vi "AIT 1553 - Parse BM Channels.vi"(6 "Bus Config Info":T12, 7 "FIFO Idx Qs":T14, 8 "error in (no error)":errorcluster, 10 "Section GUID":string, 11 "Device Reference in":T15 format="%.0x") -> (0 "error out":errorcluster, 1 "Section BaseRate":u32, 2 "HW Channel - BM Section":T1 {"Message Settings"."Driver Data"."First Word" min=8 max=31; "Message Settings"."Driver Data"."Num Bits" min=1 max=32; "Message Settings"."Driver Data"."Start Bit" min=8 max=31; "Message Settings"."Block Data Refs"."Data Reference" format="%.0x"; "Rx Com Udp Port"."Handle" format="%08x"; "Tx Com Udp Port"."Handle" format="%08x"}, 3 "Device Reference out":T15 format="%.0x")   [LabVIEW 2013]
uses:
  <vilib>/NI Veristand/Custom Device Tools/Custom Device Utility Library/Custom Device Utility Library.lvlib
  <vilib>/NI Veristand/Custom Device API/Custom Device API.lvlib
  Controls and Global/Number of Bits.ctl
  AIT 664 Custom Device.lvlib
  Controls and Global/Start Bit.ctl
  <vilib>/NI Veristand/Custom Device API/Data Reference.ctl
  <vilib>/NI Veristand/Custom Device API/Block Data Reference.ctl
  Controls and Global/Global.vi
  <vilib>/NI Veristand/Custom Device Tools/Custom Device Utility Library/NI VeriStand - Search for Item by GUID.vi
  RT Controls/AIT 664 - RT Message Settings.ctl
  RT Controls/AIT 664 - RT Hardware Channel.ctl
  RT Controls/AIT 664 - Driver Data.ctl
  RT Controls/AIT 1553 - Bus Section.ctl
  System Explorer/Controls/664 - Sampling Type.ctl
  <userlib>/ARINC 664/AIT 664 Controls/General/Message Port Type.ctl
  <userlib>/ARINC 664/AIT 664 API.lvlib
  <userlib>/ARINC 664/AIT 664 Controls/General/Direction.ctl
  <userlib>/ARINC 664/AIT 664 Controls/General/Message Port.ctl
  <vilib>/NI Veristand/Custom Device API/Custom Device Item Ref.ctl
  RT Controls/FIFO Index Queues.ctl
  RT Controls/AIT 1553 - Hardware Type.ctl
  RT Controls/AIT 1553 - Board Config Info.ctl
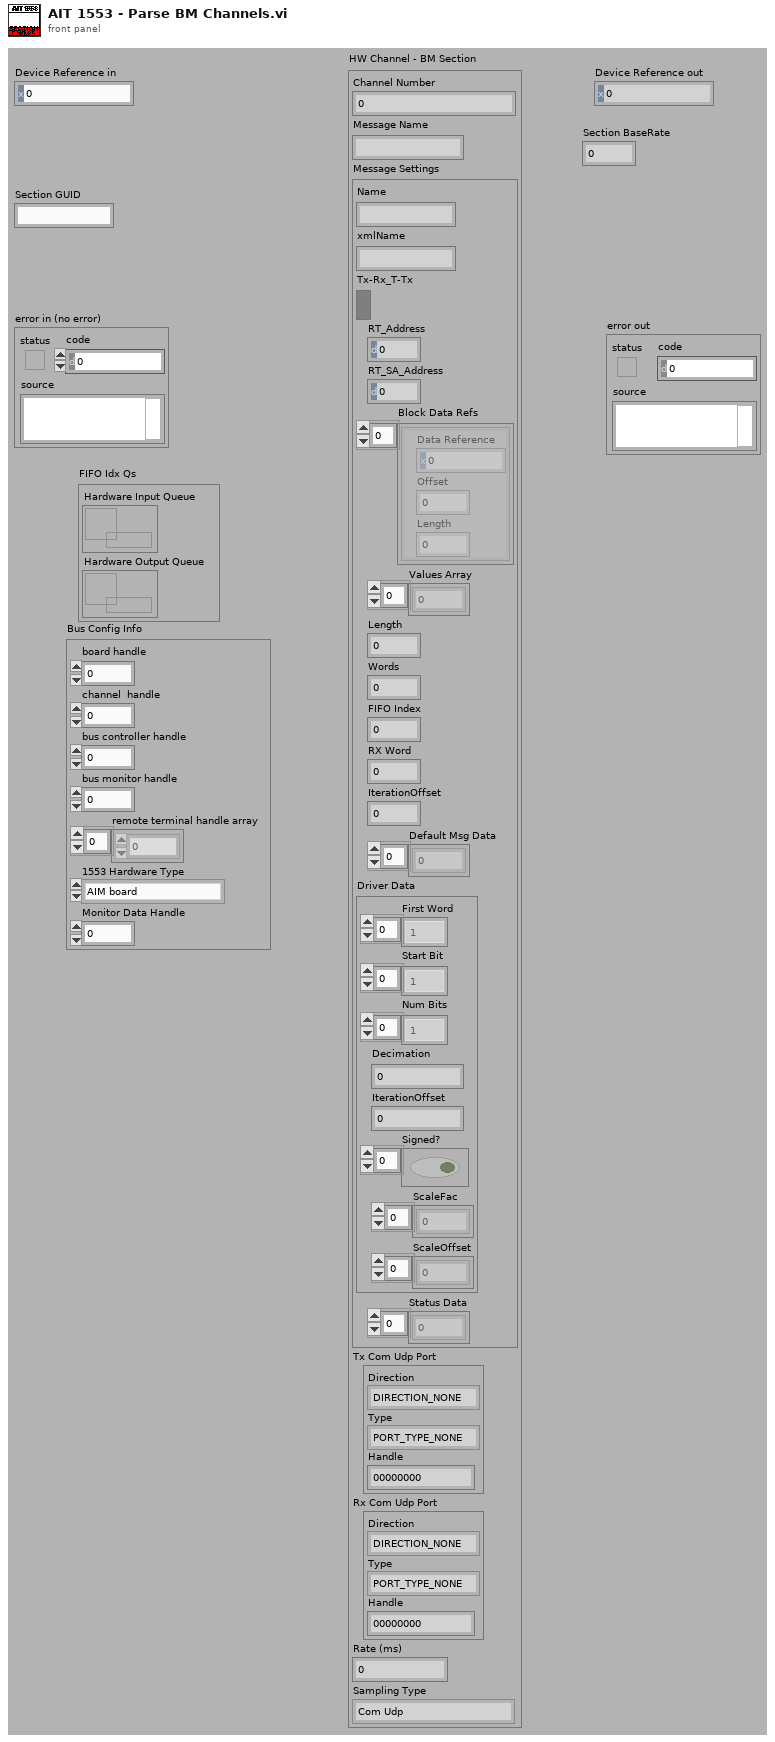
[diagram p1: front panel]
types:
  T1 = typedef "AIT 664 Custom Device.lvlib/AIT 664 - RT Hardware Channel.ctl" = cluster{"Channel Number":u16, "Message Name":string, "Message Settings":T2, "Tx Com Udp Port":T8, "Rx Com Udp Port":T8, "Rate (ms)":u32, "Sampling Type":T11}
  T2 = typedef "AIT 664 Custom Device.lvlib/AIT 664 - RT Message Settings.ctl" = cluster{"Name":string, "xmlName":string, "Tx-Rx_T-Tx":bool, "RT_Address":u8, "RT_SA_Address":u8, "Block Data Refs":T3[], "Values Array":dbl[], "Length":i32, "Words":i32, "FIFO Index":i32, "RX Word":u32, "IterationOffset":i32, "Default Msg Data":u8[], "Driver Data":T5, "Status Data":u32[]}
  T3 = typedef "Custom Device API.lvlib/Block Data Reference.ctl" = cluster{"Data Reference":T4, "Offset":i32, "Length":i32}
  T4 = typedef "Custom Device API.lvlib/Data Reference.ctl" = i32
  T5 = typedef "AIT 664 Custom Device.lvlib/AIT 664 - Driver Data.ctl" = cluster{"First Word":T6[], "Start Bit":T6[], "Num Bits":T7[], "Decimation":i32, "IterationOffset":i32, "Signed?":bool[], "ScaleFac":dbl[], "ScaleOffset":dbl[]}
  T6 = typedef "AIT 664 Custom Device.lvlib/Start Bit.ctl" = i32
  T7 = typedef "AIT 664 Custom Device.lvlib/Number of Bits.ctl" = i32
  T8 = typedef "AIT 664 API.lvlib/Message Port.ctl" = cluster{"Direction":T9, "Type":T10, "Handle":u64}
  T9 = typedef "AIT 664 API.lvlib/Direction.ctl" = enum16{"DIRECTION_NONE", "DIRECTION_TX", "DIRECTION_RX"}
  T10 = typedef "AIT 664 API.lvlib/Message Port Type.ctl" = enum16{"PORT_TYPE_NONE", "COM_UDP", "SAP_UDP", "SAP_IP", "SAP_MAC", "COTS_MAC", "COTS_MAC_RAW"}
  T11 = typedef "AIT 664 Custom Device.lvlib/664 - Sampling Type.ctl" = enum16{"Com Udp", "Com Udp Queuing", "Sap Udp", "Sap Ip", "Sap Mac", "Unknown"}
  T12 = typedef "AIT 1553 - Board Config Info.ctl" = cluster{"board handle":u32, "channel  handle":u32, "bus controller handle":u32, "bus monitor handle":u32, "remote terminal handle array":u32[], "1553 Hardware Type":T13, "Monitor Data Handle":u32}
  T13 = typedef "AIT 1553 - Hardware Type.ctl" = enum16{"AIM board", "AIT Board"}
  T14 = typedef "AIT 664 Custom Device.lvlib/FIFO Index Queues.ctl" = cluster{"Hardware Input Queue":refnum<queue>, "Hardware Output Queue":refnum<queue>}
  T15 = typedef "Custom Device API.lvlib/Custom Device Item Ref.ctl" = u64
  T16 = typedef "AIT 1553 - Bus Section.ctl" = enum16{"BC", "BM", "RT"}
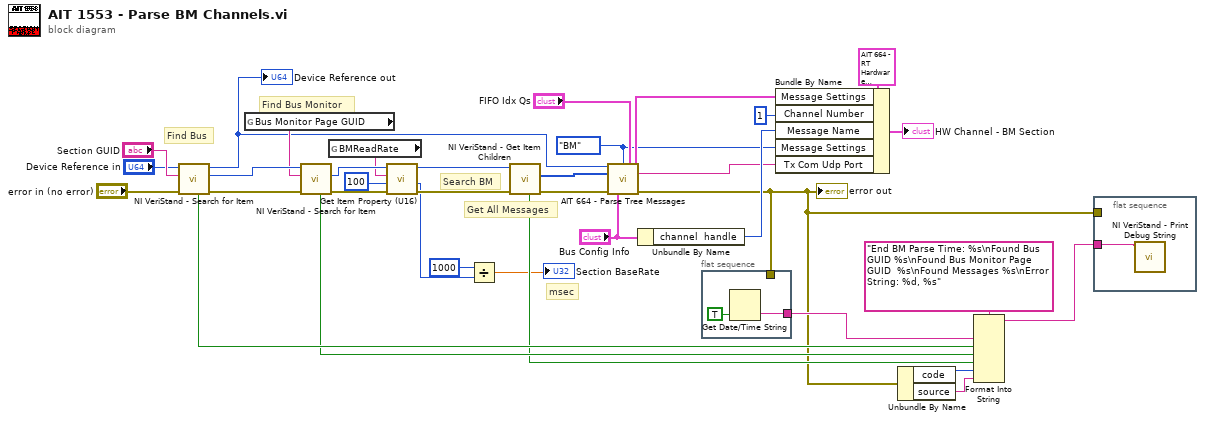
[diagram p0: block diagram]
diagram:
  w15 = AIT_1553_-_Bus_Section."BM" ("Bus Section")
  # "msec"
  # "Find Bus Monitor"
  # "Find Bus"
  # "Get All Messages"
  # "Search BM"
  n1 = call-poly <vilib>:"NI VeriStand - Search for Item.vi"("error in"="error in (no error)", "Item GUID"="Section GUID", "Section Ref in"="Device Reference in") -> ("error out"=w26:errorcluster, "Item Ref"=w27:T15, "Section Ref out"=w16:T15, "Found"=w23:bool)  [unwired: 5 in]
  "Device Reference out" <- w16
  n2 = global read "Global.vi" "Bus Monitor Page GUID"() -> (w25:string)
  n3 = call-poly <vilib>:"NI VeriStand - Search for Item.vi"("error in"=w26, "Item GUID"=w25, "Section Ref in"=w27) -> ("error out"=w9:errorcluster, "Item Ref"=w8:T15, "Found"=w22:bool)  [unwired: 5 in, 1 out]
  n4 = global read "Global.vi" "BMReadRate"() -> (w1:string)
  n5 = call <vilib>:"Get Item Property (U16).vi"("error in (no error)"=w9, "Default Value"=u16 100 ("Section BaseRate"), "Property Name"=w1, "Item Ref in"=w8) -> ("error out"=w6:errorcluster, "Value"=w3:u16, "Item Ref out"=w7:T15)  [unwired: 4 in, 1 out]
  n6 = Divide(x=u16 1000 ("Section BaseRate"), y=w3) -> (x/y=→"Section BaseRate":dbl)
  n7 = call <vilib>:"NI VeriStand - Get Item Children.vi"("error in (no error)"=w6, "Item Ref in"=w7) -> ("error out"=w20:errorcluster, "Child Refs"=w33:T15[], "Found"=w18:bool)  [unwired: 6 in, 1 out]
  n8 = call "AIT 664 - Parse Tree Messages.vi"("Custom Device Ref"=w16, 2:w15, "FIFO Idx Qs"="FIFO Idx Qs", "Message Ref"=w33, "error out"=w20, 12:"Bus Config Info") -> ("Message Settings"=w30:T2, "Message Name"=w14:string, "error out"=w12:errorcluster)  [unwired: 7 in]
  "error out" <- w12
  n9 = Unbundle By Name("Bus Config Info") -> ("channel  handle"=w28:u32)
  n10 = flat-sequence {
    tunnel: [w38] -> w13
    tunnel: w12 -> [_]
    frame #0 {
      n11 = Get Date/Time String(want seconds? (F)=TRUE) -> (time string=w38:string)  [unwired: 2 in, 1 out]
    }
  }
  n12 = Bundle By Name(cluster=T1 {"Channel Number"=0, "Message Name"="", "Message Settings"={"Name"="", "xmlName"="", "Tx-Rx_T-Tx"=FALSE, "RT_Address"=0, "RT_SA_Address"=0, "Block Data Refs"=[], "Values Array"=[], "Length"=0, "Words"=0, "FIFO Index"=0, "RX Word"=0, "IterationOffset"=0, "Default Msg Data"=[], "Driver Data"={"First Word"=[], "Start Bit"=[], "Num Bits"=[], "Decimation"=0, "IterationOffset"=0, "Signed?"=[], "ScaleFac"=[], "ScaleOffset"=[]}, "Status Data"=[]}, "Tx Com Udp Port"={"Direction"=enum."DIRECTION_NONE", "Type"=enum."PORT_TYPE_NONE", "Handle"=0}, "Rx Com Udp Port"={"Direction"=enum."DIRECTION_NONE", "Type"=enum."PORT_TYPE_NONE", "Handle"=0}, "Rate (ms)"=0, "Sampling Type"=enum."Com Udp"} ("HW Channel"), "Message Settings"=w30, "Channel Number"=u16 1 ("channel #"), "Message Name"=w28, "Message Settings"=w15, "Tx Com Udp Port"=w14) -> (→"HW Channel - BM Section":T1)
  n13 = Unbundle By Name(w12) -> ("code"=w19:i32, "source"=w11:string)
  n14 = Format Into String(format string="End BM Parse Time: %s\nFound Bus GUID %s\nFound Bus Monitor Page GUID  %s\nFound Messages %s\nError String: %d, %s", w13, w23, w22, w18, w19, w11) -> (resulting string=w24:string)  [unwired: 2 in, 1 out]
  n15 = flat-sequence {
    tunnel: w24 -> [w39]
    tunnel: w12 -> [_]
    frame #0 {
      n16 = call <vilib>:"NI VeriStand - Print Debug String.vi"("Message"=w39) -> ()  [unwired: 10 in, 1 out]
    }
  }
